vi "Write Actor DVR.vi"(10 "Actor DVR":refnum<data-value>, 11 "Actor in":refnum<class "Actor.lvclass">) -> (3 "Actor out":refnum<class "Actor.lvclass">)   [LabVIEW 2020, in "jettl.lvlib" / "Actor.lvclass"]
uses:
  Actor.lvclass
  Msg/Msg.lvclass
  Msg Set.ctl
  jettl.lvlib
  Actor.ctl
  Refs/Refs.lvclass
  Msgs.ctl
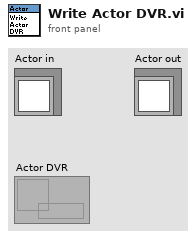
[diagram p1: front panel]
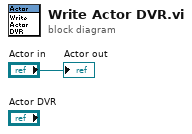
[diagram p0: block diagram]
diagram:
  "Actor out" <- "Actor in"
